vi "加1.vi"(8 "error in (no error)":errorcluster, 11 "基本数据类型 in":refnum<class "基本数据类型.lvclass">) -> (0 "error out":errorcluster, 3 "基本数据类型 out":refnum<class "基本数据类型.lvclass">)   [LabVIEW 2021, in "基本数据类型.lvclass"]
doc: "本VI是为《我和LabVIEW》一书编写的示例。\n关于本书的介绍请参考网页：\nhttp://ruanqizhen.spaces.live.com/blog/cns!5852D4F797C53FB6!4310.entry"
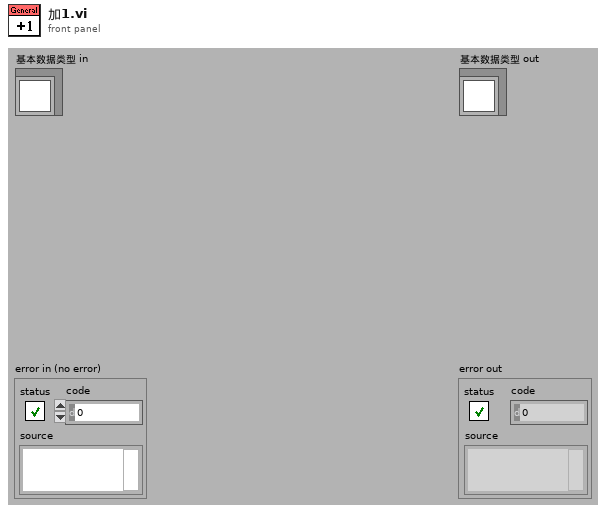
[diagram p1: front panel]
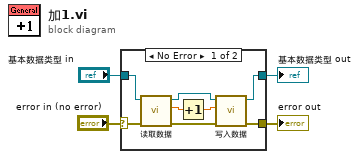
[diagram p0: block diagram]
diagram:
  n1 = case shown="No Error" "error in (no error)" {
    selector: "error in (no error)" -> [w7 w14]
    tunnel: [w5 w14] -> w3
    tunnel: [w8 w13] -> w1
    tunnel: "基本数据类型 in" -> [w9 w13]
    frame No Error {
      n2 = call-dynamic "读取数据.vi"("error in (no error)"=w7, "基本数据类型.lvclass in"=w9) -> ("error out"=w6:errorcluster, "数据"=w11:dbl, "基本数据类型.lvclass out"=w12:refnum<class "基本数据类型.lvclass">)  [unwired: 7 out]
      n3 = Increment(x=w11) -> (x+1=w10:dbl)
      n4 = call-dynamic "写入数据.vi"("error in (no error)"=w6, "数据"=w10, "基本数据类型.lvclass in"=w12) -> ("error out"=w5:errorcluster, "基本数据类型.lvclass out"=w8:refnum<class "基本数据类型.lvclass">)  [unwired: 7 out]
    }
    frame Error {
    }
  }
  "error out" <- w3
  "基本数据类型 out" <- w1
